vi "Page_Windows_Security_Read.vi"(6 "output cluster":T1, 8 "error in (no error)":errorcluster, 11 "IB_MSI in":refnum<class "IB_MSI.lvclass">) -> (0 "error out":errorcluster, 3 "IB_MSI out":refnum<class "IB_MSI.lvclass">)   [LabVIEW 2020, in "IB_MSI.lvclass"]
uses:
  <vilib>/AppBuilder/IB_Classes/MSI/IB_MSI.lvclass
  <vilib>/AppBuilder/IB_Classes/MSI/IB_MSI.lvclass/IB_MSI.ctl
  <vilib>/AppBuilder/CodeSignAPI/CodeSignAPI.lvlib
  <resource>/Framework/Providers/Common/provcom_StringGlobals.vi
  <resource>/Framework/Providers/Builds/AppBuilder/AB_UI_Page_Windows_Security_References.ctl
  <resource>/Framework/Providers/Common/provcom_BrowseProjectFile.ctl
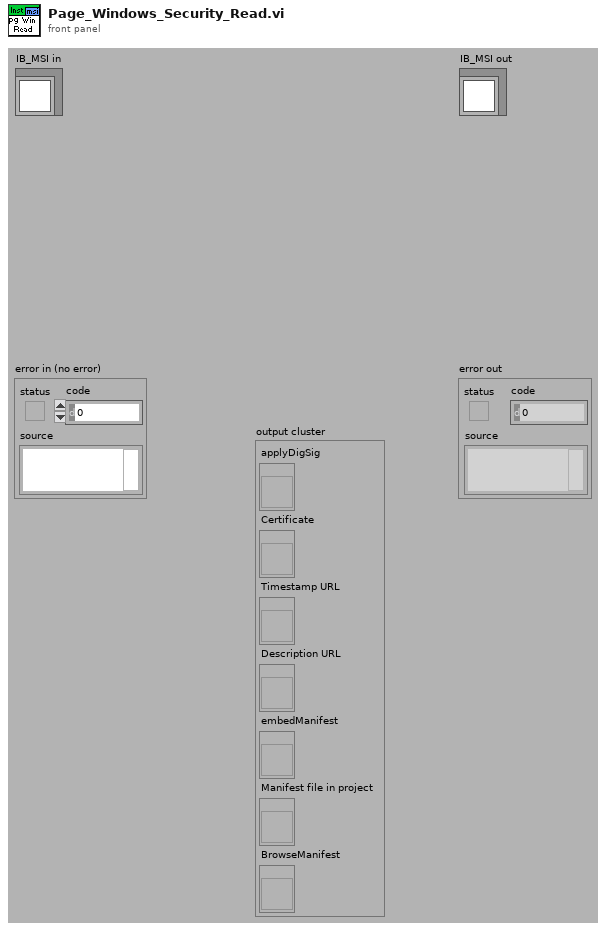
[diagram p1: front panel]
types:
  T1 = typedef "AB_UI_Page_Windows_Security_References.ctl" = cluster{"applyDigSig":refnum<vi>, "Certificate":refnum<vi>, "Timestamp URL":refnum<vi>, "Description URL":refnum<vi>, "embedManifest":refnum<vi>, "Manifest file in project":refnum<vi>, "BrowseManifest":refnum<vi>}
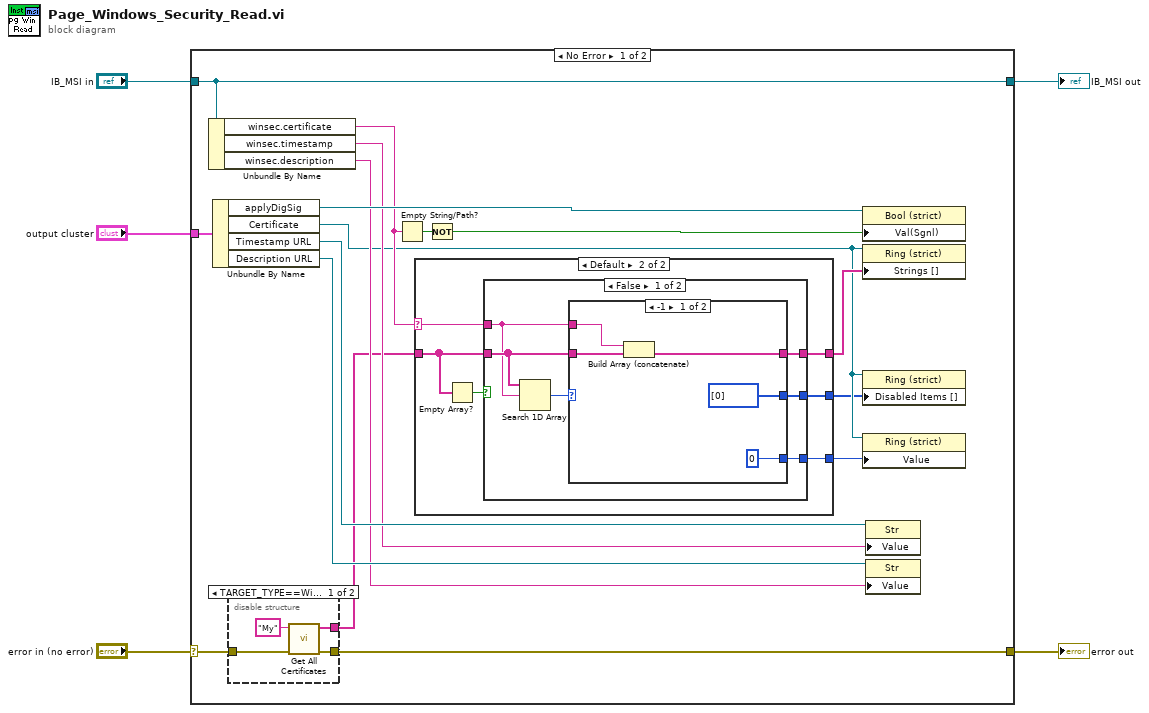
[diagram p0: block diagram]
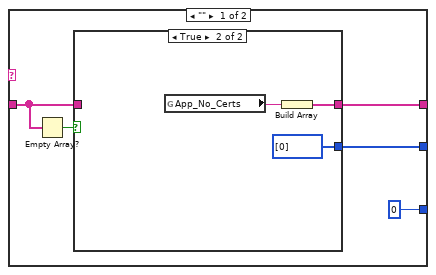
[diagram p3: hidden frame]
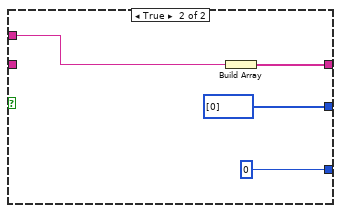
[diagram p6: hidden frame]
diagram:
  n1 = case shown="No Error" "error in (no error)" {
    selector: "error in (no error)" -> [w22 w60]
    tunnel: "IB_MSI in" -> [w15 w61]
    tunnel: [w15 w61] -> w4
    tunnel: [w21 w60] -> w2
    tunnel: "output cluster" -> [w6 _]
    frame No Error {
      n2 = Unbundle By Name(w15) -> ("winsec.certificate"=w12:string, "winsec.timestamp"=w18:string, "winsec.description"=w16:string)
      n3 = Unbundle By Name(w6) -> ("applyDigSig"=w20:refnum<vi>, "Certificate"=w8:refnum<vi>, "Timestamp URL"=w19:refnum<vi>, "Description URL"=w17:refnum<vi>)
      n4 = disable-structure shown="TARGET_TYPE==Windows" {
        disable-tunnel: w22 -> [w25 w27]
        disable-tunnel: [w24 w27] -> w21
        disable-tunnel: [w23 _] -> w11
        frame condition #0 (active) {
          n5 = call <vilib>:"Get All Certificates.vi"("error in (no error)"=w25, "store"="My") -> ("error out"=w24:errorcluster, "Certificates"=w23:string[])  [unwired: 8 out]
        }
        frame condition #1 {
        }
      }
      n6 = Empty String/Path?(string/path=w12) -> (empty?=w14:bool)
      n7 = case shown="Default" w12 {
        selector: w12 -> [_ w39]
        tunnel: w11 -> [w31 w41]
        tunnel: [w30 w38] -> w10
        tunnel: [u16 0 ("Value") w40] -> w9
        tunnel: [w28 w37] -> w7
        frame "" {
          n8 = Empty Array?(array=w31) -> (empty?=w32:bool)
          n9 = case shown="True" w32 {
            tunnel: [w33 w35] -> w30
            tunnel: w31 -> [w33 _]
            tunnel: [_ i32[] [0]] -> w28
            frame False {
            }
            frame True {
              n10 = global read "provcom_StringGlobals.vi" "App_No_Certs"() -> (w36:string)
              n11 = Build Array(w36) -> (w35:string[])
            }
          }
        }
        frame Default {
          n12 = Empty Array?(array=w41) -> (empty?=w42:bool)
          n13 = case shown="False" w42 {
            tunnel: [w46 w59] -> w38
            tunnel: w41 -> [w47 _]
            tunnel: [w43 0] -> w40
            tunnel: w39 -> [w45 w57]
            tunnel: [w44 i32[] [0]] -> w37
            frame False {
              n14 = Search 1D Array(1D array=w47, element=w45) -> (index of element=w48:i32)  [unwired: 1 out]
              n15 = case shown="-1" w48 {
                selector: w48 -> [_ w54]
                tunnel: [w49 w55] -> w46
                tunnel: w47 -> [w53 w55]
                tunnel: w45 -> [w52 _]
                tunnel: [i32[] [0] _] -> w44
                tunnel: [0 w54] -> w43
                frame -1 {
                  n16 = Build Array (concatenate)(w52, w53) -> (w49:string[])
                }
                frame Default {
                }
              }
            }
            frame True {
              n17 = Build Array(w57) -> (w59:string[])
            }
          }
        }
      }
      n18 = Not(x=w14) -> (.not. x?=w13:bool)
      n19 = property class="Bool (strict)"(reference=w20, "Val(Sgnl)"=w13) -> ()  [unwired: 1 in, 2 out]
      n20 = property class="Ring (strict)"(reference=w8, "Strings []"=w10) -> ()  [unwired: 1 in, 2 out]
      n21 = property class="Ring (strict)"(reference=w8, "Disabled Items []"=w7) -> ()  [unwired: 1 in, 2 out]
      n22 = property class="Ring (strict)"(reference=w8, "Value"=w9) -> ()  [unwired: 1 in, 2 out]
      n23 = property class="Str"(reference=w19, "Value"=w18) -> ()  [unwired: 1 in, 2 out]
      n24 = property class="Str"(reference=w17, "Value"=w16) -> ()  [unwired: 1 in, 2 out]
    }
    frame Error {
    }
  }
  "error out" <- w2
  "IB_MSI out" <- w4
